vi "Convert Cfg Cluster 2 to 3.vi"(10 "Tool Face Ref":sgl=1.0, 11 "Tool Config Cluster_v2":T1={"Tool Type"=0, "Tool SN"=0, "Tool Block"={"Encoder Size"=0, "Encoder Scale"=0, "Encoder Offset"=0, "MaxEncoder"=0, "MinEncoder"=0, "Start Delay"=0.0}, "Motor Block"={"MinMotor Speed"=0, "MaxMotor Speed"=0, "Homing Speed"=90, "Jog Speed"=90, "Inspect Speed"=90, "VBlk Speed"=90, "CleaningPos"=0, "Safe Zone"=0, "Has Motor"=FALSE, "Use Home Index"=FALSE}, "Verification Block"={"Angle"=90.0, "FlankLength1"=0.0, "FlankLength2"=0.0, "Location"=0.0, "Serial Number"=0}, "Probe Block"={"nProbes"=0, "Probe Param Array"=[]}}) -> (3 "Tool Config Cluster_v3":T9={"Tool Type"=0, "Tool SN"=0, "Tool Block"={"Encoder Size"=0, "Encoder Scale"=0, "Encoder Offset"=0, "MaxEncoder"=0, "MinEncoder"=0, "Start Delay"=0.0, "Tool Face Ref"=0.0}, "Motor Block"={"MinMotor Speed"=0, "MaxMotor Speed"=0, "Homing Speed"=90, "Jog Speed"=90, "Inspect Speed"=90, "VBlk Speed"=90, "CleaningPos"=0, "Safe Zone"=0, "Has Motor"=FALSE, "Use Home Index"=FALSE}, "Verification Block"={"Angle"=90.0, "FlankLength1"=0.0, "FlankLength2"=0.0, "Location"=0.0, "Serial Number"=0}, "Probe Block"={"nProbes"=0, "Probe Param Array"=[]}} {"Probe Block"."Probe Param Array"."Sensor Block"."SensorCfgParams Array"."CalibrCoefArray" format="%#.12g"})   [LabVIEW 2015, in "Tool Cfg.lvlib"]
uses:
  Tool Cfg.lvlib
  _Configuration Cluster_v3--typedef.ctl
  _Tool Block Cluster_v3--typedef.ctl
  _Motor Block Cluster_v2--typedef.ctl
  _Verification Blk Cluster--typedef.ctl
  _ProbeConfigParams Cluster--typedef.ctl
  _Sensor Block Cluster--typedef.ctl
  _SensorConfigParams Cluster--typedef.ctl
  _Configuration Cluster_v2--typedef.ctl
  _Tool Block Cluster--typedef.ctl
  _Probe Block Cluster--typedef.ctl
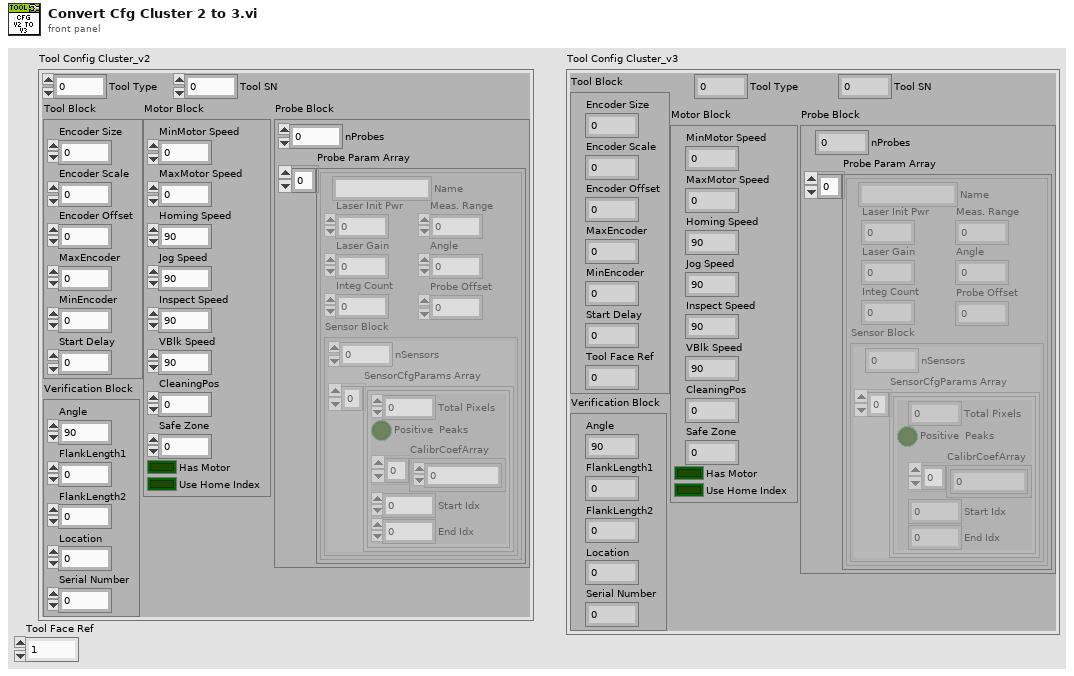
[diagram p1: front panel]
types:
  T1 = typedef "Tool Cfg.lvlib/_Configuration Cluster_v2--typedef.ctl" = cluster{"Tool Type":u16, "Tool SN":u16, "Tool Block":T2, "Motor Block":T3, "Verification Block":T4, "Probe Block":T5}
  T2 = typedef "Tool Cfg.lvlib/_Tool Block Cluster--typedef.ctl" = cluster{"Encoder Size":u16, "Encoder Scale":u32, "Encoder Offset":i32, "MaxEncoder":i32, "MinEncoder":i32, "Start Delay":sgl}
  T3 = typedef "Tool Cfg.lvlib/_Motor Block Cluster_v2--typedef.ctl" = cluster{"MinMotor Speed":u16, "MaxMotor Speed":u16, "Homing Speed":u16, "Jog Speed":u16, "Inspect Speed":u16, "VBlk Speed":u16, "CleaningPos":i32, "Safe Zone":i32, "Has Motor":bool, "Use Home Index":bool}
  T4 = typedef "Tool Cfg.lvlib/_Verification Blk Cluster--typedef.ctl" = cluster{"Angle":sgl, "FlankLength1":sgl, "FlankLength2":sgl, "Location":sgl, "Serial Number":u16}
  T5 = typedef "Tool Cfg.lvlib/_Probe Block Cluster--typedef.ctl" = cluster{"nProbes":u16, "Probe Param Array":T6[]}
  T6 = typedef "Tool Cfg.lvlib/_ProbeConfigParams Cluster--typedef.ctl" = cluster{"Name":string, "Laser Init Pwr":u16, "Laser Gain":u8, "Integ Count":u16, "Meas. Range":sgl, "Angle":sgl, "Probe Offset":sgl, "Sensor Block":T7}
  T7 = typedef "Tool Cfg.lvlib/_Sensor Block Cluster--typedef.ctl" = cluster{"nSensors":u16, "SensorCfgParams Array":T8[]}
  T8 = typedef "Tool Cfg.lvlib/_SensorConfigParams Cluster--typedef.ctl" = cluster{"Total Pixels":u16, "Positive  Peaks":bool, "CalibrCoefArray":dbl[], "Start Idx":u16, "End Idx":u16}
  T9 = typedef "Tool Cfg.lvlib/_Configuration Cluster_v3--typedef.ctl" = cluster{"Tool Type":u16, "Tool SN":u16, "Tool Block":T10, "Motor Block":T3, "Verification Block":T4, "Probe Block":cluster{"nProbes":u16, "Probe Param Array":T6[]}}
  T10 = typedef "Tool Cfg.lvlib/_Tool Block Cluster_v3--typedef.ctl" = cluster{"Encoder Size":u16, "Encoder Scale":u32, "Encoder Offset":i32, "MaxEncoder":i32, "MinEncoder":i32, "Start Delay":sgl, "Tool Face Ref":sgl}
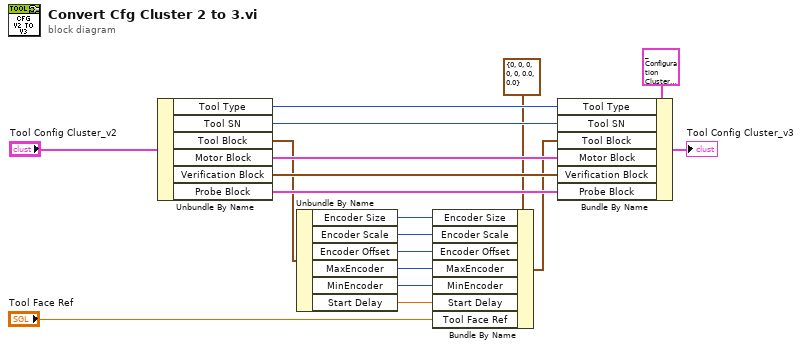
[diagram p0: block diagram]
diagram:
  n1 = Unbundle By Name("Tool Config Cluster_v2") -> ("Tool Type"=w18:u16, "Tool SN"=w17:u16, "Tool Block"=w10:T2, "Motor Block"=w11:T3, "Verification Block"=w16:T4, "Probe Block"=w15:T5)
  n2 = Unbundle By Name(w10) -> ("Encoder Size"=w3:u16, "Encoder Scale"=w4:u32, "Encoder Offset"=w5:i32, "MaxEncoder"=w6:i32, "MinEncoder"=w7:i32, "Start Delay"=w8:sgl)
  n3 = Bundle By Name(cluster=T10 {"Encoder Size"=0, "Encoder Scale"=0, "Encoder Offset"=0, "MaxEncoder"=0, "MinEncoder"=0, "Start Delay"=0.0, "Tool Face Ref"=0.0} ("_Tool Block Cluster_v3--typedef"), "Encoder Size"=w3, "Encoder Scale"=w4, "Encoder Offset"=w5, "MaxEncoder"=w6, "MinEncoder"=w7, "Start Delay"=w8, "Tool Face Ref"="Tool Face Ref") -> (w1:T10)
  n4 = Bundle By Name(cluster=T9 {"Tool Type"=0, "Tool SN"=0, "Tool Block"={"Encoder Size"=0, "Encoder Scale"=0, "Encoder Offset"=0, "MaxEncoder"=0, "MinEncoder"=0, "Start Delay"=0.0, "Tool Face Ref"=0.0}, "Motor Block"={"MinMotor Speed"=0, "MaxMotor Speed"=0, "Homing Speed"=90, "Jog Speed"=90, "Inspect Speed"=90, "VBlk Speed"=90, "CleaningPos"=0, "Safe Zone"=0, "Has Motor"=FALSE, "Use Home Index"=FALSE}, "Verification Block"={"Angle"=90.0, "FlankLength1"=0.0, "FlankLength2"=0.0, "Location"=0.0, "Serial Number"=0}, "Probe Block"={"nProbes"=0, "Probe Param Array"=[]}} ("_Tool Config Cluster_v3--typedef"), "Tool Type"=w18, "Tool SN"=w17, "Tool Block"=w1, "Motor Block"=w11, "Verification Block"=w16, "Probe Block"=w15) -> (→"Tool Config Cluster_v3":T9)
